vi "decode-data.vi"() -> ()   [LabVIEW 2010]
panel:
  out "数据输出字符串":string
  out "输出类别字符串":string
  in  "输入字符串":string="060001010234781216"
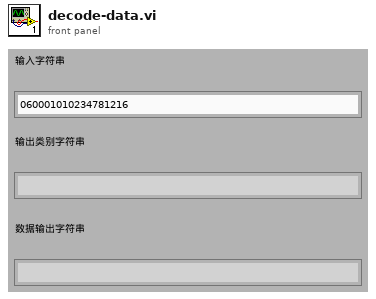
[diagram p1: front panel]
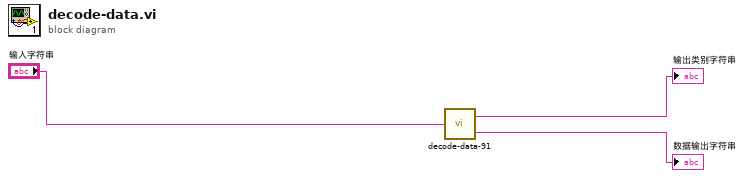
[diagram p0: block diagram]
diagram:
  n1 = call "decode-data-91.vi"("输入字符串"="输入字符串") -> ("数据字符串"=→"数据输出字符串":string, "类型字符串"=→"输出类别字符串":string)
